vi "Global - UI Stream and Variable Connections.vi"() -> ()   [LabVIEW 2018]
uses:
  support/Message Queue/Message Cluster.ctl
  controls/Variable References.ctl
  support/Message Queue/Message Queue.lvlib
panel:
  in  "Variable References":T1
  in  "RT Message Stream":refnum<k21>
  in  "UI Command Stream":refnum<k21>
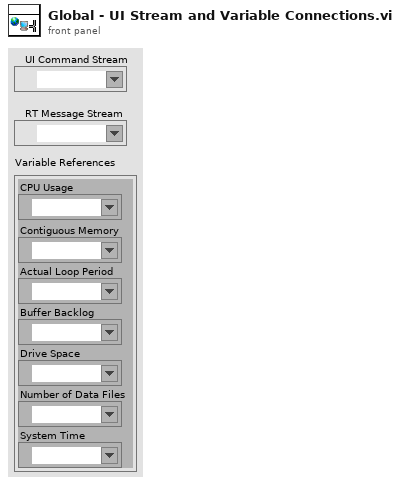
[diagram p1: front panel]
types:
  T1 = typedef "Variable References.ctl" = cluster{"CPU Usage":refnum<k21>, "Contiguous Memory":refnum<k21>, "Actual Loop Period":refnum<k21>, "Buffer Backlog":refnum<k21>, "Drive Space":refnum<k21>, "Number of Data Files":refnum<k21>, "System Time":refnum<k21>}
diagram:
